vi "Actor API Type.vi"(11 "Template Artifex in":refnum<class "Template.lvclass">) -> (2 "Actor API Type":refnum<class "Actor API.lvclass">)   [LabVIEW 2020, in "Artifex Template.lvlib" / "Template.lvclass"]
uses:
  Template.lvclass
  Template API/Template API.lvclass
  Artifex/Actor Proxy/Actor API.lvclass
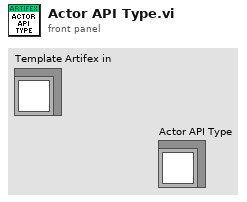
[diagram p1: front panel]
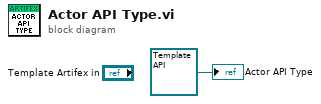
[diagram p0: block diagram]
diagram:
  "Actor API Type" <- refnum<class "Template API.lvclass"> refnum ("Artifex Template.lvlib:Template API.lvclass")
